vi "setExternalTrigger.vi"() -> ()   [LabVIEW 2012]
uses:
  hidapi_32bits.dll
panel:
  out "Result":i32
  in  "signalFrontMode":u8
  in  "enableMode":u8
  # "enableMode:\n0 - trigger disabled\n1 - trigger enabled\n2 - one time trigger\n\ntriggerFront:\n0 - trigger disabled\n1 - front rising\n2 - front falling\n3 - both rising and fall"
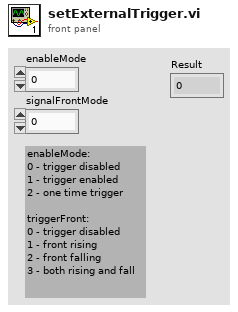
[diagram p1: front panel]
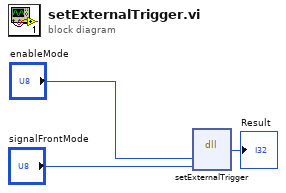
[diagram p0: block diagram]
diagram:
  n1 = dll-call lib="C:/All_Data/mikrocont/Project1/New_controller__Jan_2015/LabView_Aug_2015/hidapi_32bits.dll" fn="setExternalTrigger"("enableMode"="enableMode", "signalFrontMode"="signalFrontMode") -> ("return type"=→"Result":i32)  [unwired: 5 in, 2 out]
